vi "API_DB.ExecuteSQlCommand.vi"(6 "Timeout (ms)":u32, 7 "Wait (F)":bool, 8 "error in (no error)":errorcluster, 10 "SQLCommand":string, 11 "DLP2 in":refnum<class "DLP2.lvclass">) -> (0 "error out":errorcluster, 2 "Return Value":variant, 3 "DLP2 out":refnum<class "DLP2.lvclass">)   [LabVIEW 2022 SP3, in "DLP2.lvclass"]
doc: "Developed by Kevin Thompson\nkevin@thompsonengineering.net\n\nCopyright 2018\nThompson Engineering, LLC"
uses:
  DLP2.lvclass
  DataTypes/AsynCmd_Temp01--enum.ctl
  DLP2.lvclass/DLP2.ctl
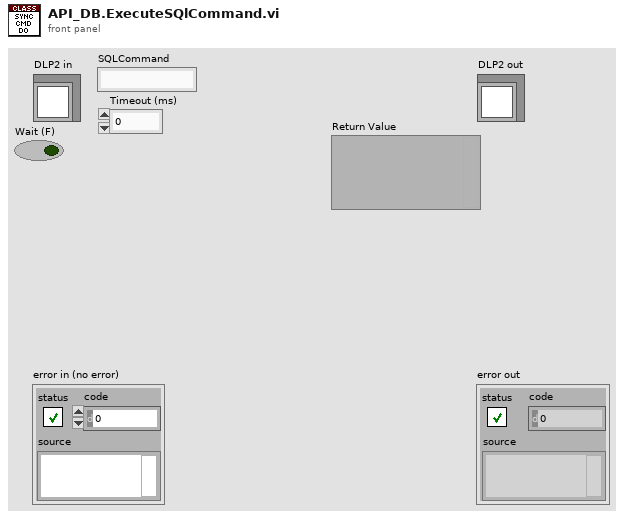
[diagram p1: front panel]
types:
  T1 = typedef "DLP2.lvclass/AsynCmd_Temp01--enum.ctl" = enum16{"DB.DeleteRecord", "DB.UpdateRecord", "DB.InsertRecord", "DB.SelectRecord", "DB.ExecuteSQLCommand", "DB.FindFirstSlot", "DB.GenericSQLQuery"}
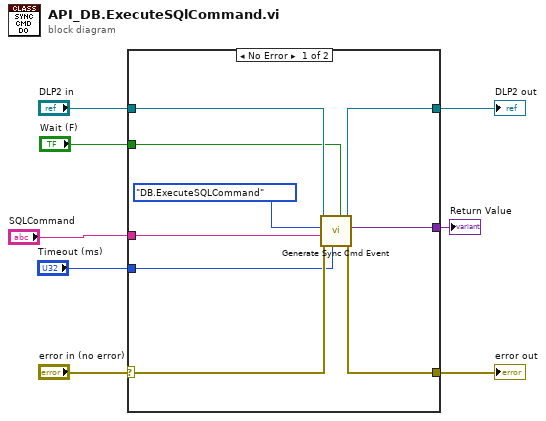
[diagram p0: block diagram]
diagram:
  n1 = case shown="No Error" "error in (no error)" {
    selector: "error in (no error)" -> [w15 w19]
    tunnel: [w14 w19] -> w7
    tunnel: [w16 w18] -> w5
    tunnel: "DLP2 in" -> [w17 w18]
    tunnel: "SQLCommand" -> [w12 _]
    tunnel: "Wait (F)" -> [w11 _]
    tunnel: "Timeout (ms)" -> [w10 _]
    tunnel: [w9 _] -> w1
    frame No Error {
      n2 = call "Generate Sync Cmd Event.vi"("Wait (F)"=w11, "Timeout (ms)"=w10, "error in (no error)"=w15, "vData"=w12, "AsyncCmd"=AsynCmd_Temp01--enum."DB.ExecuteSQLCommand", "DLP2 in"=w17) -> ("error out"=w14:errorcluster, "Return Value"=w9:variant, "DLP2 out"=w16:refnum<class "DLP2.lvclass">)  [unwired: 3 in]
    }
    frame Error {
    }
  }
  "error out" <- w7
  "DLP2 out" <- w5
  "Return Value" <- w1
